vi "PluginsLoaderCommander_ReadCommand.vi"(8 "error in (no error)":errorcluster, 9 "timeout in ms (-1)":i32, 11 "PluginsLoaderCommander in":refnum<class "PluginsLoaderCommander.lvclass">) -> (0 "error out":errorcluster, 1 "Data":variant, 2 "Command":T1, 3 "PluginsLoaderCommander out":refnum<class "PluginsLoaderCommander.lvclass">)   [LabVIEW 2014, in "PluginsThread.lvlib" / "PluginsLoaderCommander.lvclass"]
uses:
  PluginsLoaderCommander.lvclass
  PluginsLoaderCommander_Command.ctl
  PluginsLoaderCommander.lvclass/PluginsLoaderCommander.ctl
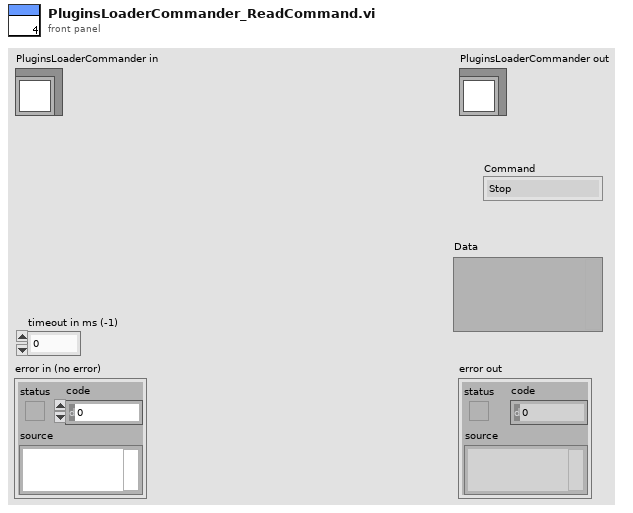
[diagram p1: front panel]
types:
  T1 = typedef "PluginsThread.lvlib/PluginsLoaderCommander.lvclass/PluginsLoaderCommander_Command.ctl" = enum16{"Stop", "Timeout"}
  T2 = typedef "PluginsThread.lvlib/PluginsLoaderCommander.lvclass/PluginsLoaderCommander_CommandData.ctl" = cluster{"Command":T1, "Data":variant}
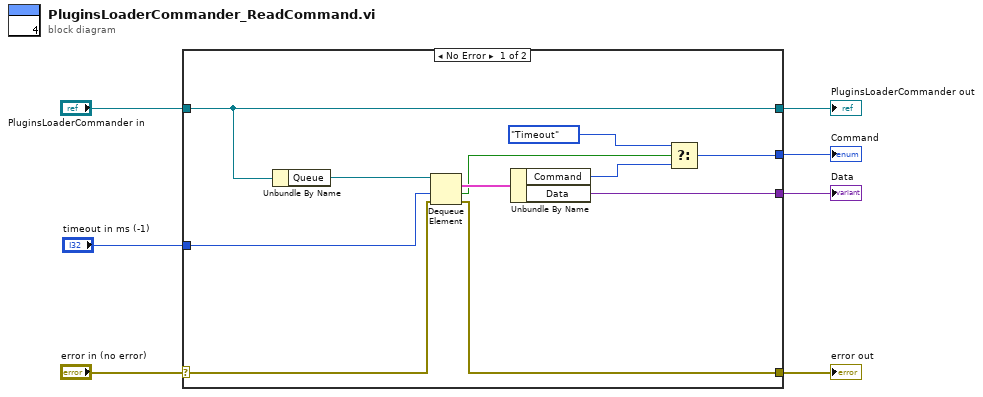
[diagram p0: block diagram]
diagram:
  n1 = case shown="No Error" "error in (no error)" {
    selector: "error in (no error)" -> [w16 w20]
    tunnel: [w15 w20] -> w6
    tunnel: [w18 w19] -> w4
    tunnel: "PluginsLoaderCommander in" -> [w18 w19]
    tunnel: "timeout in ms (-1)" -> [w14 _]
    tunnel: [w9 _] -> w2
    tunnel: [w12 _] -> w1
    frame No Error {
      n2 = Unbundle By Name(w18) -> ("Queue"=w17:refnum<queue>)
      n3 = Dequeue Element(queue=w17, timeout in ms (-1)=w14, error in (no error)=w16) -> (element=w13:T2, timed out?=w11:bool, error out=w15:errorcluster)  [unwired: 1 out]
      n4 = Unbundle By Name(w13) -> ("Command"=w10:T1, "Data"=w12:variant)
      n5 = Select(t=PluginsLoaderCommander_Command."Timeout", s=w11, f=w10) -> (s? t:f=w9:T1)
    }
    frame Error {
    }
  }
  "error out" <- w6
  "PluginsLoaderCommander out" <- w4
  "Command" <- w2
  "Data" <- w1
